vi "Dictionary Test - 005.vi"(8 "error in (no error)":errorcluster) -> (0 "error out":errorcluster, 2 "pass":bool)   [LabVIEW 2009]
uses:
  source/library/Dictionary Update/Dictionary Update (by value).vi
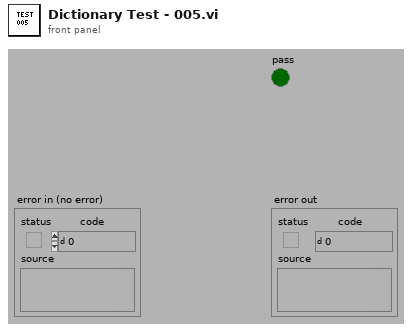
[diagram p1: front panel]
types:
  T1 = typedef "Dictionary Object RefNum.ctl" = refnum<k1>
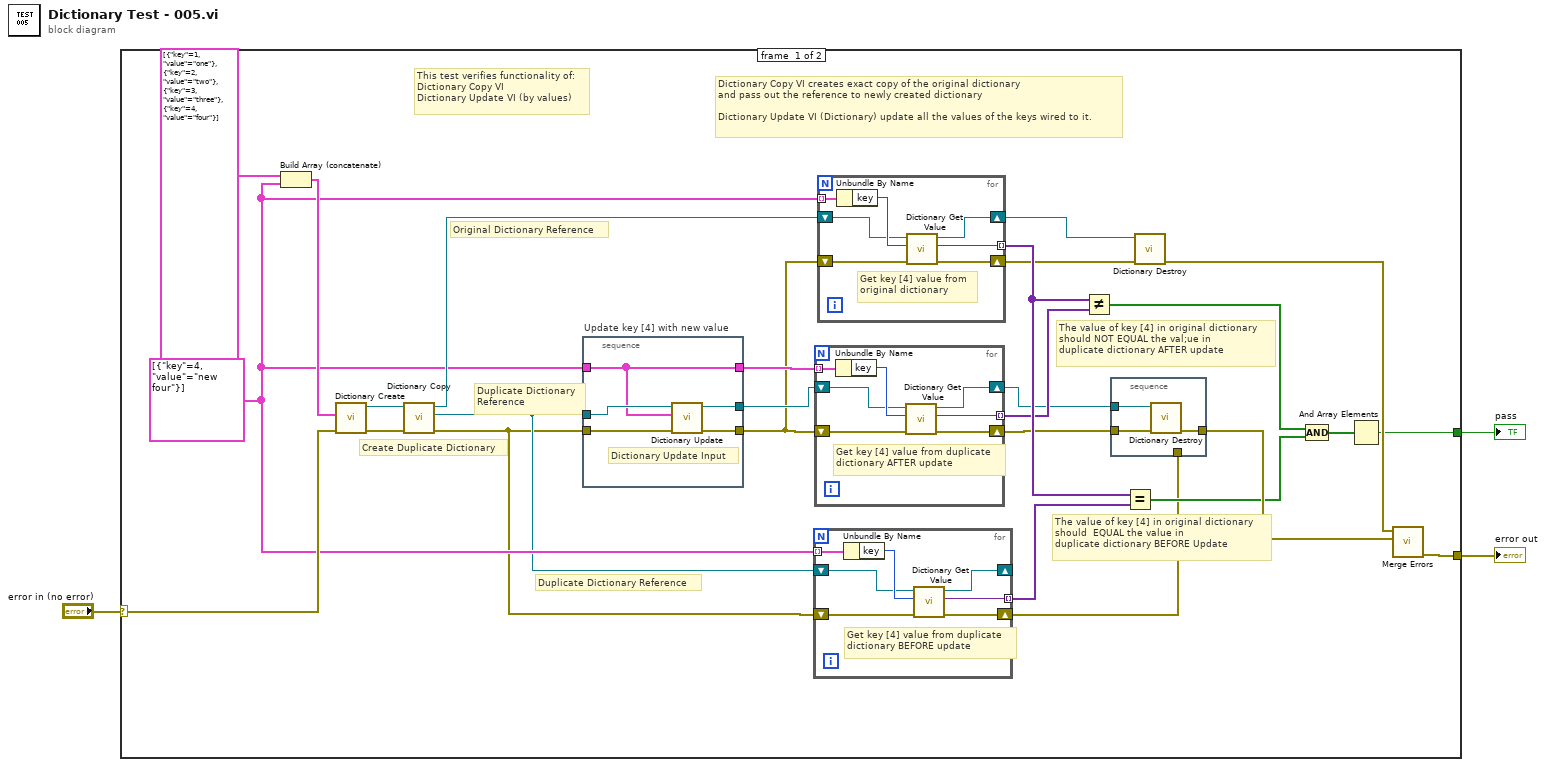
[diagram p0: block diagram]
diagram:
  n1 = case shown="No Error" "error in (no error)" {
    selector: "error in (no error)" -> [w30 w60]
    tunnel: [w26 w60] -> w2
    tunnel: [w5 _] -> w1
    frame #0 {
      w15 = cluster{"key":i32, "value":string}[] [{"key"=4, "value"="new four"}]
      # "The value of key [4] in original dictionary\nshould  EQUAL the value in \nduplicate dictionary BEFORE Update"
      # "The value of key [4] in original dictionary\nshould NOT EQUAL the val;ue in \nduplicate dictionary AFTER update"
      # "Duplicate Dictionary Reference"
      # "Duplicate Dictionary\nReference"
      # "Original Dictionary Reference"
      # "Create Duplicate Dictionary"
      # "Dictionary Copy VI creates exact copy of the original dictionary \nand pass out the reference to newly created dictionary\n\nDictionary Update VI (Dictionary) update all the values of the keys wired to it."
      # "This test verifies functionality of:\nDictionary Copy VI\nDictionary Update VI (by values)"
      n2 = Build Array (concatenate)(cluster{"key":i32, "value":string}[] [{"key"=1, "value"="one"}, {"key"=2, "value"="two"}, {"key"=3, "value"="three"}, {"key"=4, "value"="four"}] ("dictionary with updates"), w15) -> (w23:cluster{"key":i32, "value":string}[])
      n3 = call "Dictionary Create.vi"("error in (no error)"=w30, "initial dictionary (empty)"=w23) -> ("error out"=w27:errorcluster, "dictionary out"=w28:T1)  [unwired: 8 in]
      n4 = call "Dictionary Copy.vi"("error in (no error)"=w27, "dictionary"=w28) -> ("error out"=w13:errorcluster, "new dictionary out"=w14:T1, "dictionary out"=w17:T1)  [unwired: 7 in]
      n5 = stacked-sequence "Update key [4] with new value" {
        tunnel: [w59] -> w10
        tunnel: [w55] -> w11
        tunnel: w14 -> [w58]
        tunnel: w15 -> [w55]
        tunnel: [w57] -> w9
        tunnel: w13 -> [w56]
        frame #0 {
          # "Dictionary Update Input"
          n6 = call-poly "Dictionary Update.vi"("error in (no error)"=w56, "dictionary with updates"=w55, "dictionary"=w58) -> ("error out"=w57:errorcluster, "dictionary out"=w59:T1)  [unwired: 6 in, 1 out]
        }
      }
      n7 = for {
        tunnel: [w47] -> w12 mode=indexing
        tunnel: w15 -> [w46] mode=indexing
        shift-right: [w44] -> _
        shift-left: w14 -> [w43]
        shift-right: [w42] -> w4
        shift-left: w13 -> [w41]
        # "Get key [4] value from duplicate\ndictionary BEFORE update"
        n8 = Unbundle By Name(w46) -> ("key"=w45:i32)
        n9 = call "Dictionary Get Value.vi"("error in"=w41, "key"=w45, "dictionary"=w43) -> ("error out"=w42:errorcluster, "value"=w47:variant, "dictionary out"=w44:T1)  [unwired: 5 in, 1 out]
      }
      n10 = for {
        tunnel: [w40] -> w8 mode=indexing
        tunnel: w11 -> [w39] mode=indexing
        shift-right: [w37] -> w7
        shift-left: w10 -> [w36]
        shift-right: [w35] -> w6
        shift-left: w9 -> [w34]
        # "Get key [4] value from duplicate\ndictionary AFTER update"
        n11 = Unbundle By Name(w39) -> ("key"=w38:i32)
        n12 = call "Dictionary Get Value.vi"("error in"=w34, "key"=w38, "dictionary"=w36) -> ("error out"=w35:errorcluster, "value"=w40:variant, "dictionary out"=w37:T1)  [unwired: 5 in, 1 out]
      }
      n13 = for {
        tunnel: [w54] -> w21 mode=indexing
        tunnel: w15 -> [w53] mode=indexing
        shift-right: [w51] -> w18
        shift-left: w17 -> [w50]
        shift-right: [w49] -> w16
        shift-left: w9 -> [w48]
        # "Get key [4] value from\noriginal dictionary"
        n14 = Unbundle By Name(w53) -> ("key"=w52:i32)
        n15 = call "Dictionary Get Value.vi"("error in"=w48, "key"=w52, "dictionary"=w50) -> ("error out"=w49:errorcluster, "value"=w54:variant, "dictionary out"=w51:T1)  [unwired: 5 in, 1 out]
      }
      n16 = Not Equal?(x=w21, y=w8) -> (x != y?=w22:bool[])
      n17 = stacked-sequence {
        tunnel: [w33] -> w24
        tunnel: w7 -> [w32]
        tunnel: w6 -> [w31]
        tunnel: w4 -> [_]
        frame #0 {
          n18 = call "Dictionary Destroy.vi"("error in (no error)"=w31, "dictionary"=w32) -> ("error out"=w33:errorcluster)  [unwired: 9 in]
        }
      }
      n19 = Equal?(x=w21, y=w12) -> (x = y?=w19:bool[])
      n20 = call "Dictionary Destroy.vi"("error in (no error)"=w16, "dictionary"=w18) -> ("error out"=w25:errorcluster)  [unwired: 9 in]
      n21 = Compound Arithmetic op=AND(w22, w19) -> (w20:bool[])
      n22 = And Array Elements(Boolean array=w20) -> (logical AND=w5:bool)
      n23 = call <vilib>:"Merge Errors.vi"("error in 2 (no error)"=w24, "error in 1 (no error)"=w25) -> ("error out"=w26:errorcluster)  [unwired: 5 in]
    }
    frame #1 {
    }
  }
  "pass" <- w1
  "error out" <- w2
